vi "Read Gif Images.vi"(8 "error in (no error)":errorcluster, 11 "Gif Parent in":refnum<class "GIF Parent.lvclass">) -> (0 "error out":errorcluster, 2 "Gif Images":picture[](array[picture]), 3 "Gif Parent out":refnum<class "GIF Parent.lvclass">)   [LabVIEW 2021, in "GIF Parent.lvclass"]
doc: "read the image array for the gif file"
uses:
  GIF Parent.lvclass
  GIF Parent.lvclass/GIF Parent.ctl
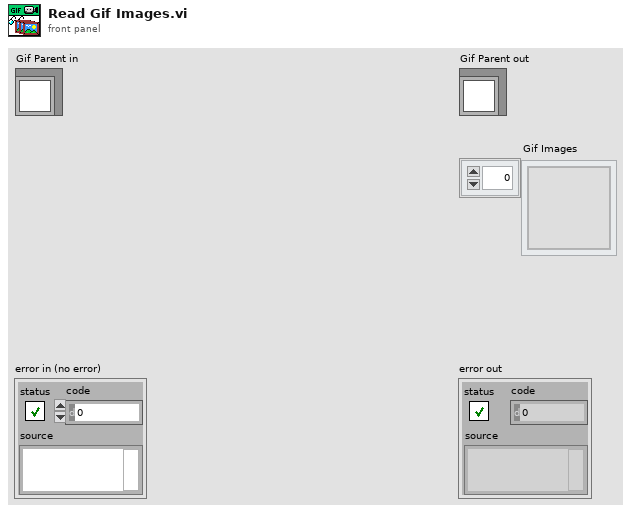
[diagram p1: front panel]
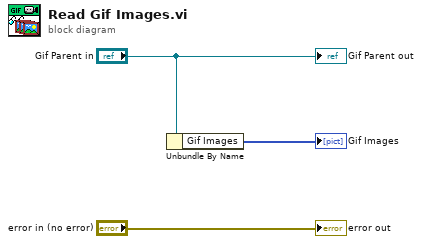
[diagram p0: block diagram]
diagram:
  n1 = Unbundle By Name("Gif Parent in") -> ("Gif Images"=→"Gif Images":picture[])
  "error out" <- "error in (no error)"
  "Gif Parent out" <- "Gif Parent in"
